vi "Main - Timer (SubVI).vi"(6 "Enum":enum16{"Write", "Read"}(ring)=enum."Read", 8 "error in (no error)":errorcluster, 11 "Elapsed Time Target":dbl=12.0 format="%0.8f") -> (0 "error out":errorcluster, 1 "Elapsed TimeText":string, 2 "Time has Elapsed":bool, 3 "Elapsed Time":dbl format="%0.2f")   [LabVIEW 2019]
uses:
  Controls/FGV States.ctl
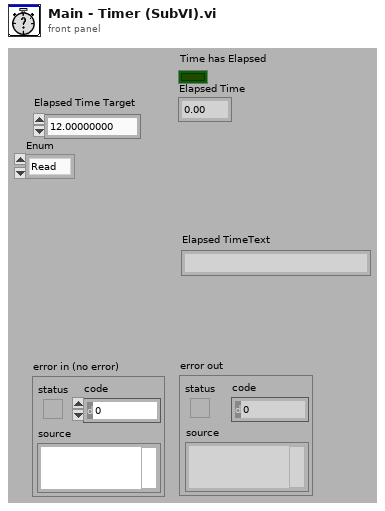
[diagram p1: front panel]
types:
  T1 = typedef "FGV States.ctl" = enum16{"Read", "Write"}
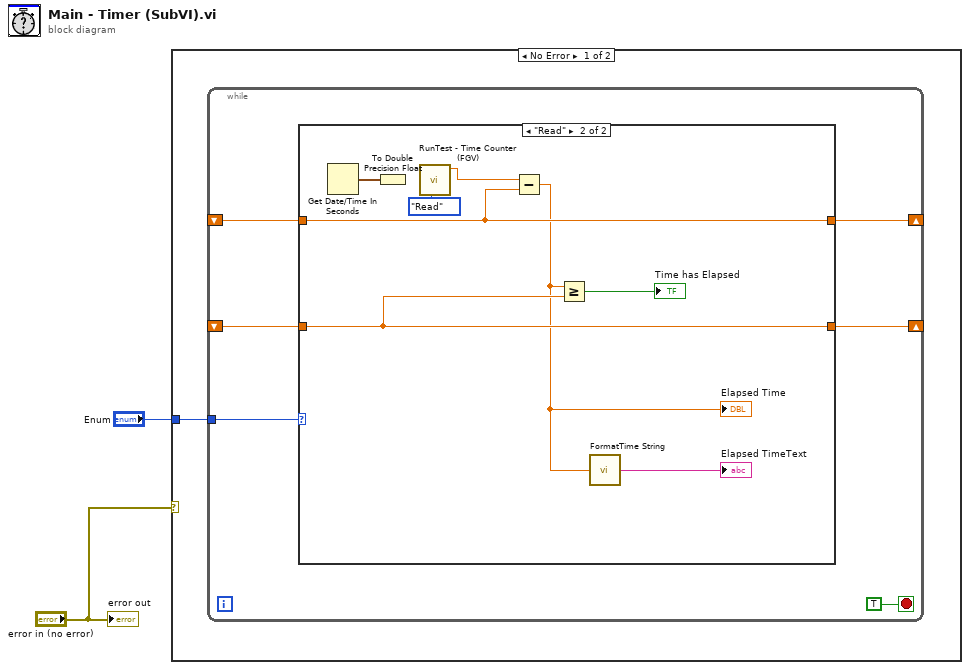
[diagram p0: block diagram]
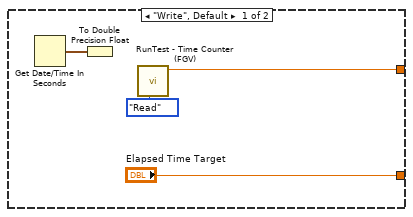
[diagram p2: hidden frame]
diagram:
  n1 = case shown="No Error" "error in (no error)" {
    tunnel: "Enum" -> [w3 _]
    frame No Error {
      n2 = while {
        tunnel: w3 -> [w8]
        shift-right: [w7] -> _
        shift-left: _ -> [w5]
        shift-right: [w6] -> _
        shift-left: _ -> [w4]
        stop <- TRUE stop-if-true
        n3 = case shown="\"Read\"" w8 {
          tunnel: [w10 w20] -> w7
          tunnel: ["Elapsed Time Target" w19] -> w6
          tunnel: w5 -> [_ w20]
          tunnel: w4 -> [_ w19]
          frame "Write", Default {
            n4 = Get Date/Time In Seconds() -> (seconds since 1Jan1904=w13:timestamp)
            n5 = To Double Precision Float(number=w13) -> ()  [unwired: 1 out]
            n6 = call "RunTest - Time Counter (FGV).vi"("Action"=FGV_States."Read") -> ("Calib out"=w10:dbl)  [unwired: 9 in, 1 out]
          }
          frame "Read" {
            n7 = Get Date/Time In Seconds() -> (seconds since 1Jan1904=w21:timestamp)
            n8 = To Double Precision Float(number=w21) -> ()  [unwired: 1 out]
            n9 = call "RunTest - Time Counter (FGV).vi"("Action"=FGV_States."Read") -> ("Calib out"=w14:dbl)  [unwired: 9 in, 1 out]
            n10 = Subtract(x=w14, y=w20) -> (x-y=w16:dbl)
            "Elapsed Time" <- w16
            n11 = Greater Or Equal?(x=w16, y=w19) -> (x >= y?=→"Time has Elapsed":bool)
            n12 = call <vilib>:"FormatTime String.vi"("Numeric"=w16) -> ("Date/Time"=→"Elapsed TimeText":string)
          }
        }
      }
    }
    frame Error {
    }
  }
  "error out" <- "error in (no error)"
